vi "test-chassis-speed_DUP_DELETE.vi"() -> ()   [LabVIEW 2019]
uses:
  <vilib>/Rock Robotics/WPI/ThirdParty/JAS_Junk/TrajLib/Rotation_GetCos.vi
  <vilib>/Rock Robotics/WPI/ThirdParty/JAS_Junk/TrajLib/Rotation_GetSin.vi
  <vilib>/Rock Robotics/WPI/ThirdParty/JAS_Junk/TrajLib/ChassisSpeeds_New.vi
  <vilib>/Rock Robotics/WPI/ThirdParty/JAS_Junk/TrajLib/Trajectory_Library.lvlib
panel:
  out "T0 -- Ras/sec -- 0":dbl
  out "T0 -- y -- 0":dbl
  out "T0 -- X -- 0":dbl
  # "Chassis Speed Test"
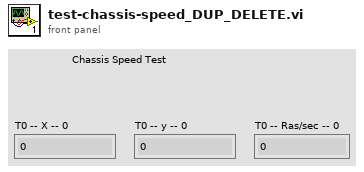
[diagram p1: front panel]
types:
  T1 = typedef "Trajectory_Library.lvlib/ROTATION2D.ctl" = cluster{"VALUE":dbl, "COS":dbl, "SIN":dbl}
  T2 = typedef "Trajectory_Library.lvlib/CHASSIS_SPEEDS.ctl" = cluster{"vX":dbl, "vY":dbl, "vOmega":dbl}
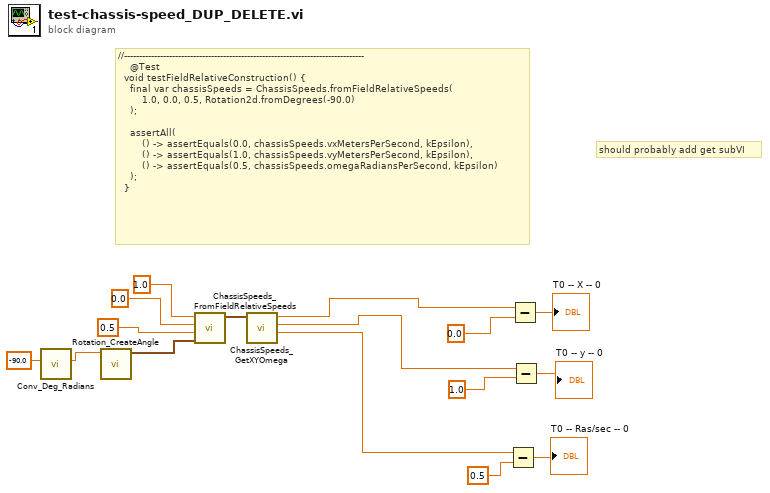
[diagram p0: block diagram]
diagram:
  # "should probably add get subVI"
  # "//--------------------------------------------------------------------------------\n    @Test\n  void testFieldRelativeConstruction() {\n    final var chassisSpeeds = ChassisSpeeds.fromFieldRelativeSpeeds(\n        1.0, 0.0, 0.5, Rotation2d.fromDegrees(-90.0)\n    );\n\n    assertAll(\n        () -> assertEquals(0.0, chassisSpeeds.vxMetersPerSecond, kEpsilon),\n        () -> assertEquals(1.0, chassisSpeeds.vyMetersPerSecond, kEpsilon),\n        () -> assertEquals(0.5, chassisSpeeds.omegaRadiansPerSecond, kEpsilon)\n    );\n  }"
  n1 = call <vilib>:"Conv_Deg_Radians.vi"("Degress"=-90.0) -> ("Radians"=w11:dbl)  [unwired: 10 in]
  n2 = call <vilib>:"Rotation_CreateAngle.vi"("Angle"=w11) -> ("ROTATION"=w8:T1)  [unwired: 10 in]
  n3 = call <vilib>:"ChassisSpeeds_FromFieldRelativeSpeeds.vi"("RobotAngle"=w8, "Omega"=0.5, "vY"=0.0, "vX"=1.0) -> ("CHASSIS"=w4:T2)  [unwired: 7 in]
  n4 = call <vilib>:"ChassisSpeeds_GetXYOmega.vi"("CHASSIS"=w4) -> ("vAngular"=w1:dbl, "vY"=w2:dbl, "vX"=w3:dbl)  [unwired: 8 in]
  n5 = Subtract(x=w1, y=0.5) -> (x-y=→"T0 -- Ras/sec -- 0":dbl)
  n6 = Subtract(x=w3, y=0.0) -> (x-y=→"T0 -- X -- 0":dbl)
  n7 = Subtract(x=w2, y=1.0) -> (x-y=→"T0 -- y -- 0":dbl)
